vi "hdf5 image file ref FGV.vi"(6 "Camera name":string, 8 "error in (no error)":errorcluster, 9 "module path in":path, 10 "command":enum16{"set", "get"}(ring)=enum."get", 11 "Python session":refnum<k35>) -> (0 "error out":errorcluster, 1 "module path":path, 3 "Python session":refnum<k35>, 4 "Camera name out":string)   [LabVIEW 2020]
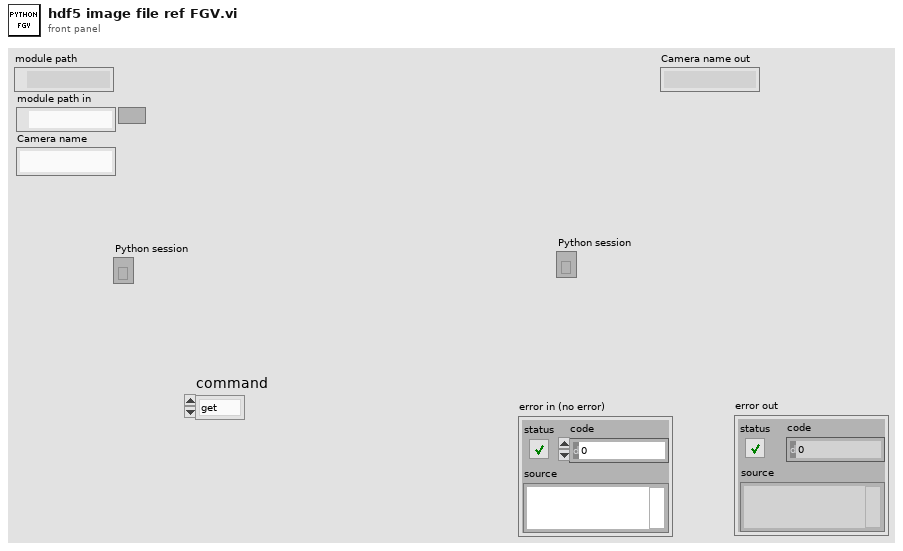
[diagram p1: front panel]
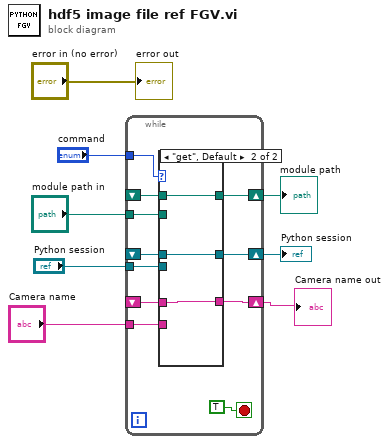
[diagram p0: block diagram]
diagram:
  n1 = while {
    shift-right: [w16] -> w5
    shift-left: _ -> [w17]
    tunnel: "command" -> [w18]
    tunnel: "Python session" -> [w15]
    tunnel: "module path in" -> [w13]
    shift-right: [w14] -> w3
    shift-left: _ -> [w12]
    shift-right: [w10] -> w1
    shift-left: _ -> [w11]
    tunnel: "Camera name" -> [w9]
    stop <- TRUE stop-if-true
    n2 = case shown="\"get\", Default" w18 {
      tunnel: w17 -> [_ w25]
      tunnel: [w22 w25] -> w16
      tunnel: w15 -> [w22 _]
      tunnel: [w21 w24] -> w14
      tunnel: w13 -> [w21 _]
      tunnel: w12 -> [_ w24]
      tunnel: [w20 w23] -> w10
      tunnel: w11 -> [_ w23]
      tunnel: w9 -> [w20 _]
      frame "set" {
      }
      frame "get", Default {
      }
    }
  }
  "Python session" <- w5
  "module path" <- w3
  "Camera name out" <- w1
  "error out" <- "error in (no error)"
